vi "ELVIS III v1.1 Stop AO Continuous.vi"(7 "Wait Until Done?":bool, 8 "error in (no error)":errorcluster, 10 "Channel Info":T1, 11 "myRIO Ref In":T2) -> (0 "error out":errorcluster, 3 "myRIO Ref Out":T2 caption="myRIO Ref In")   [LabVIEW 2021]
uses:
  <vilib>/myRIO/Common/Instrument Driver Framework/Utilities/typedefs/myRIO v1.0 Reference.ctl
  <vilib>/myRIO/Common/Instrument Driver Framework/Utilities/typedefs/Generic FPGA Reference.ctl
  <vilib>/myRIO/Common/Instrument Driver Framework/ELVIS III v1.0/AO Continuous/typedefs/AO Continuous Channel Info.ctl
  <vilib>/myRIO/Common/Instrument Driver Framework/ELVIS III v1.0/AO Block/typedefs/ELVIS III AO Block Channels FPGA Reference.ctl
  <vilib>/rvi/errors/niLvFpgaAdjustHostInterfaceError.vi
  <vilib>/rvi/interface/nirviReadWriteControl/nirviReadWriteControl.xnode
  <vilib>/rvi/interface/nirviMethod/nirviMethod.xnode
  NiFpgaLv.dll
  <vilib>/rvi/interface/Simulation/niFpgaSimulationCallBeginRW.vi
  <vilib>/FPGAPlugInAG/Dynamic/niLvFpga_StartFifo_Dynamic.vi
  <vilib>/rvi/errors/niLvFpgaMergeErrorWithErrorCode.vi
  <vilib>/FPGAPlugInAG/Dynamic/niLvFpga_StopFifo_Dynamic.vi
  <vilib>/FPGAPlugInAG/Dynamic/niLvFpga_WriteFifo_Dynamic.vi
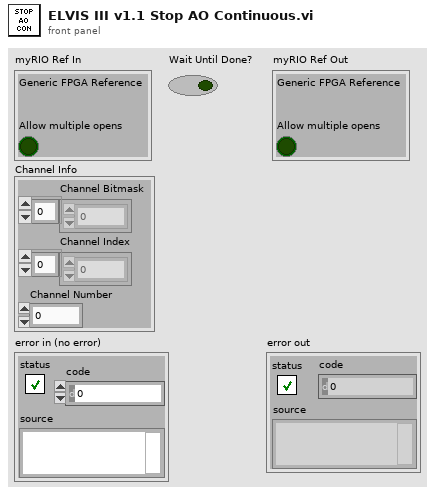
[diagram p1: front panel]
types:
  T1 = typedef "AO Continuous Channel Info.ctl" = cluster{"Channel Bitmask":u8[], "Channel Index":i32[], "Channel Number":u8}
  T2 = typedef "myRIO v1.0 Reference.ctl" = cluster{"Generic FPGA Reference":T3, "Allow multiple opens":bool}
  T3 = typedef "Generic FPGA Reference.ctl" = refnum<k20>
  T4 = typedef "ELVIS III AO Block Channels FPGA Reference.ctl" = refnum<k20>
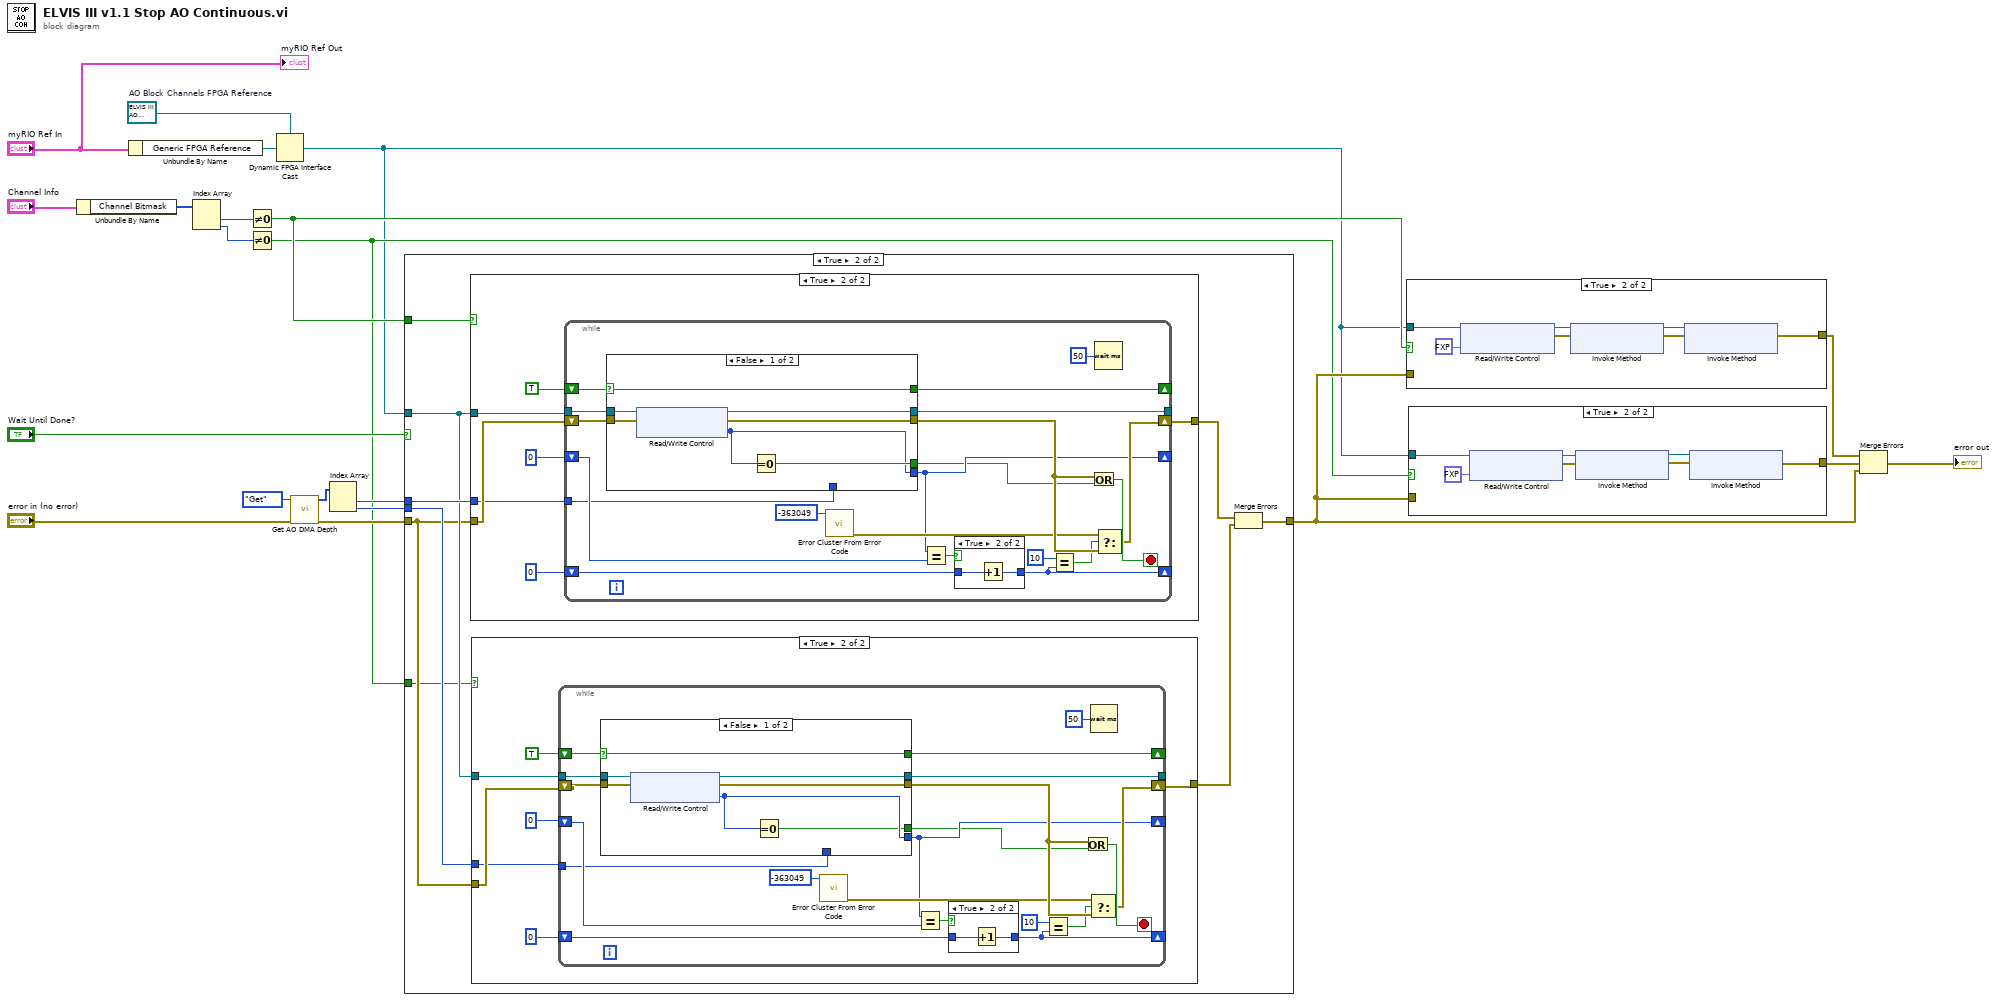
[diagram p0: block diagram]
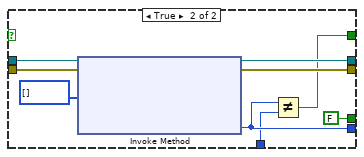
[diagram p4: hidden frame]
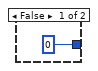
[diagram p5: hidden frame]
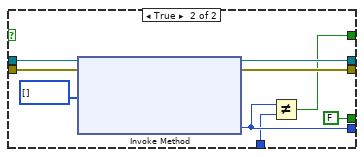
[diagram p7: hidden frame]
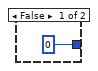
[diagram p8: hidden frame]
diagram:
  w19 = T4 refnum  # AO Block Channels FPGA Reference
  n1 = Unbundle By Name("Channel Info") -> ("Channel Bitmask"=w11:u8[])
  n2 = Unbundle By Name("myRIO Ref In") -> ("Generic FPGA Reference"=w20:T3)
  n3 = Index Array(array=w11) -> (element #1=w14:u8, element #2=w13:u8)  [unwired: 2 in]
  n4 = Not Equal To 0?(x=w14) -> (x != 0?=w3:bool)
  n5 = Not Equal To 0?(x=w13) -> (x != 0?=w2:bool)
  n6 = Dynamic FPGA Interface Cast(Session In=w19, Type=w20) -> (Session Out=w1:T4)
  n7 = call <vilib>:"Get AO DMA Depth.vi"("error in (no error)"="error in (no error)", "Action"=enum16{"Get", "Set"}."Get") -> ("error out"=w8:errorcluster, "DMA Depth Out"=w7:u32[])  [unwired: 8 in]
  n8 = Index Array(array=w7) -> (element #1=w6:u32, element #2=w4:u32)  [unwired: 2 in]
  n9 = case shown="True" "Wait Until Done?" {
    tunnel: w8 -> [w22 w27]
    tunnel: [w22 w25] -> w5
    tunnel: w1 -> [_ w28]
    tunnel: w6 -> [_ w30]
    tunnel: w4 -> [_ w29]
    tunnel: w3 -> [_ w31]
    tunnel: w2 -> [_ w26]
    frame False {
    }
    frame True {
      n10 = case shown="True" w31 {
        tunnel: w28 -> [_ w86]
        tunnel: w27 -> [w79 w85]
        tunnel: w30 -> [_ w80]
        tunnel: [w79 w82] -> w24
        frame False {
        }
        frame True {
          n11 = while {
            tunnel: w86 -> [w106]
            shift-right: [w101] -> w82
            shift-left: w85 -> [w105]
            shift-right: [w93] -> _
            shift-left: u32 0 ("Empty Elements Remaining") -> [w103]
            shift-right: [w96] -> _
            shift-left: u32 0 ("Empty Elements Remaining") -> [w97]
            tunnel: [w92] -> _
            shift-right: [w90] -> _
            shift-left: TRUE -> [w91]
            tunnel: w80 -> [w89]
            stop <- w104 stop-if-true
            n12 = case shown="False" w91 {
              selector: w91 -> [w109 _]
              tunnel: w106 -> [w113 w122]
              tunnel: w105 -> [w111 w121]
              tunnel: [w110 w120] -> w102
              tunnel: [w107 w116] -> w93
              tunnel: [w112 w118] -> w92
              tunnel: [w109 w114] -> w90
              tunnel: w89 -> [_ w115]
              tunnel: [w108 FALSE] -> w88
              frame False {
                n13 = xnode "Read/Write Control"("FPGA VI Reference In"=w113, "error in"=w111) -> ("FPGA VI Reference Out"=w112:T4, "error out"=w110:errorcluster, "AO.A.ELE_NUM"=w107:u32)
                n14 = Equal To 0?(x=w107) -> (x = 0?=w108:bool)
              }
              frame True {
                n15 = xnode "Invoke Method"("FPGA VI Reference In"=w122, "error in"=w121, "Data"=i32[] []) -> ("FPGA VI Reference Out"=w118:T4, "error out"=w120:errorcluster, "Empty Elements Remaining"=w116:u32)  [unwired: 1 in]
                n16 = Not Equal?(x=w116, y=w115) -> (x != y?=w114:bool)
              }
            }
            n17 = call <vilib>:"Error Cluster From Error Code.vi"("error code (0)"=-363049) -> ("error out"=w99:errorcluster)  [unwired: 8 in]
            n18 = Equal?(x=w93, y=w103) -> (x = y?=w98:bool)
            n19 = case shown="True" w98 {
              tunnel: w97 -> [_ w125]
              tunnel: [u32 0 w124] -> w96
              frame False {
              }
              frame True {
                n20 = Increment(x=w125) -> (x+1=w124:u32)
              }
            }
            n21 = Equal?(x=u32 10, y=w96) -> (x = y?=w94:bool)
            n22 = Or(x=w102, y=w88) -> (x .or. y?=w104:bool)
            n23 = Wait (ms)(milliseconds to wait=u32 50 ("millisecond multiple")) -> ()  [unwired: 1 out]
            n24 = Select(t=w99, s=w94, f=w102) -> (s? t:f=w101:errorcluster)
          }
        }
      }
      n25 = case shown="True" w26 {
        tunnel: w28 -> [_ w38]
        tunnel: w27 -> [w32 w37]
        tunnel: w29 -> [_ w35]
        tunnel: [w32 w33] -> w23
        frame False {
        }
        frame True {
          n26 = while {
            tunnel: w38 -> [w59]
            shift-right: [w54] -> w33
            shift-left: w37 -> [w58]
            shift-right: [w46] -> _
            shift-left: u32 0 ("Empty Elements Remaining") -> [w56]
            shift-right: [w49] -> _
            shift-left: u32 0 ("x") -> [w50]
            tunnel: [w45] -> _
            shift-right: [w43] -> _
            shift-left: TRUE -> [w44]
            tunnel: w35 -> [w42]
            stop <- w57 stop-if-true
            n27 = case shown="False" w44 {
              selector: w44 -> [w62 _]
              tunnel: w59 -> [w66 w75]
              tunnel: w58 -> [w64 w74]
              tunnel: [w63 w73] -> w55
              tunnel: [w61 w69] -> w46
              tunnel: [w65 w71] -> w45
              tunnel: [w62 w67] -> w43
              tunnel: w42 -> [_ w68]
              tunnel: [w60 FALSE] -> w41
              frame False {
                n28 = xnode "Read/Write Control"("FPGA VI Reference In"=w66, "error in"=w64) -> ("FPGA VI Reference Out"=w65:T4, "error out"=w63:errorcluster, "AO.B.ELE_NUM"=w61:u32)
                n29 = Equal To 0?(x=w61) -> (x = 0?=w60:bool)
              }
              frame True {
                n30 = xnode "Invoke Method"("FPGA VI Reference In"=w75, "error in"=w74, "Data"=i32[] []) -> ("FPGA VI Reference Out"=w71:T4, "error out"=w73:errorcluster, "Empty Elements Remaining"=w69:u32)  [unwired: 1 in]
                n31 = Not Equal?(x=w69, y=w68) -> (x != y?=w67:bool)
              }
            }
            n32 = call <vilib>:"Error Cluster From Error Code.vi"("error code (0)"=-363049) -> ("error out"=w52:errorcluster)  [unwired: 8 in]
            n33 = Equal?(x=w46, y=w56) -> (x = y?=w51:bool)
            n34 = case shown="True" w51 {
              tunnel: w50 -> [_ w78]
              tunnel: [u32 0 w77] -> w49
              frame False {
              }
              frame True {
                n35 = Increment(x=w78) -> (x+1=w77:u32)
              }
            }
            n36 = Equal?(x=u32 10, y=w49) -> (x = y?=w47:bool)
            n37 = Or(x=w55, y=w41) -> (x .or. y?=w57:bool)
            n38 = Select(t=w52, s=w47, f=w55) -> (s? t:f=w54:errorcluster)
            n39 = Wait (ms)(milliseconds to wait=u32 50 ("millisecond multiple")) -> ()  [unwired: 1 out]
          }
        }
      }
      n40 = Merge Errors(w24, w23) -> (w25:errorcluster)
    }
  }
  n41 = case shown="True" w3 {
    tunnel: w1 -> [_ w132]
    tunnel: [_ w126] -> w18
    tunnel: w5 -> [_ _]
    frame False {
    }
    frame True {
      n42 = xnode "Read/Write Control"("FPGA VI Reference In"=w132, "AO.A.DMA_ENA"=fxp<+,2,2> 0.0) -> ("FPGA VI Reference Out"=w130:T4, "error out"=w128:errorcluster)  [unwired: 1 in]
      n43 = xnode "Invoke Method"("FPGA VI Reference In"=w130, "error in"=w128) -> ("FPGA VI Reference Out"=w129:T4, "error out"=w127:errorcluster)
      n44 = xnode "Invoke Method"("FPGA VI Reference In"=w129, "error in"=w127) -> ("error out"=w126:errorcluster)  [unwired: 1 out]
    }
  }
  n45 = case shown="True" w2 {
    tunnel: w1 -> [_ w139]
    tunnel: [_ w133] -> w17
    tunnel: w5 -> [_ _]
    frame False {
    }
    frame True {
      n46 = xnode "Read/Write Control"("FPGA VI Reference In"=w139, "AO.B.DMA_ENA"=fxp<+,2,2> 0.0 ("AO.A.DMA_ENA")) -> ("FPGA VI Reference Out"=w135:T4, "error out"=w134:errorcluster)  [unwired: 1 in]
      n47 = xnode "Invoke Method"("FPGA VI Reference In"=w135, "error in"=w134) -> ("FPGA VI Reference Out"=w136:T4, "error out"=w137:errorcluster)
      n48 = xnode "Invoke Method"("FPGA VI Reference In"=w136, "error in"=w137) -> ("error out"=w133:errorcluster)  [unwired: 1 out]
    }
  }
  n49 = Merge Errors(w18, w17, w5) -> (→"error out":errorcluster)
  "myRIO Ref Out" <- "myRIO Ref In"
